vi "DCA Initialize Test.vi"(0 "Instruments to Use":T9, 1 "Files Found?":bool=TRUE, 5 "Seq Count":u32, 9 "Test Parameters In":T10={"Stimulus"={"Use Instrument"=FALSE, "Normalize"=FALSE, "Blank Screen"=FALSE, "Measurement Type"=enum."Voltage DC", "Range"=enum."Auto", "Resolution"=enum."Auto"}, "Measurement"={"Topology"=enum."PI-Network", "Lock Topology"=FALSE, "ATTN Calc"=enum."Power", "Zo"=50.0}, "Limits"=[], "Normalization"={"Normalized?"=FALSE, "Rab Value"=0.0, "Rac Value"=0.0, "Rbc Value"=0.0}}, 11 "error in (no error)":errorcluster) -> (3 "Saved Instrument Configurations":cluster{"DMM Stimulus":T6, "SWI Position":T7}, 4 "Instrument IDs":T5, 6 "Next Action":string, 10 "Test Parameters Out":T10={"Stimulus"={"Use Instrument"=FALSE, "Normalize"=FALSE, "Blank Screen"=FALSE, "Measurement Type"=enum."Voltage DC", "Range"=enum."Auto", "Resolution"=enum."Auto"}, "Measurement"={"Topology"=enum."PI-Network", "Lock Topology"=FALSE, "ATTN Calc"=enum."Power", "Zo"=50.0}, "Limits"=[], "Normalization"={"Normalized?"=FALSE, "Rab Value"=0.0, "Rac Value"=0.0, "Rbc Value"=0.0}}, 12 "Calibration":T1, 14 "Driver Refs":T4, 15 "error out":errorcluster {"code" format="%.0x"})   [LabVIEW 2011]
uses:
  TypeDefs/DCA Test Parameters.ctl
  TypeDefs/DCA Stimulus Parameters.ctl
  TypeDefs/DCA Measurement Cluster.ctl
  TypeDefs/DCA Topology.ctl
  TypeDefs/DCA Attenuation Calculation.ctl
  TypeDefs/DCA Limit.ctl
  TypeDefs/DCA Limit Quantity.ctl
  TypeDefs/DCA Limit Comparison.ctl
  TypeDefs/DCA Limit Operation.ctl
  Test Referential Limit.ctl
  TypeDefs/DCA Calibration State.ctl
  server/database/Stations/Instruments/Instrument Record.ctl
  drivers/SWI/Sea-Level/TypeDefs/Sea-Level SWI Position.ctl
  drivers/DMM/DMM Driver Ref.ctl
  drivers/SWI/SWI Driver Ref.ctl
  drivers/DMM/DMM Command.ctl
  drivers/SWI/SWI Command.ctl
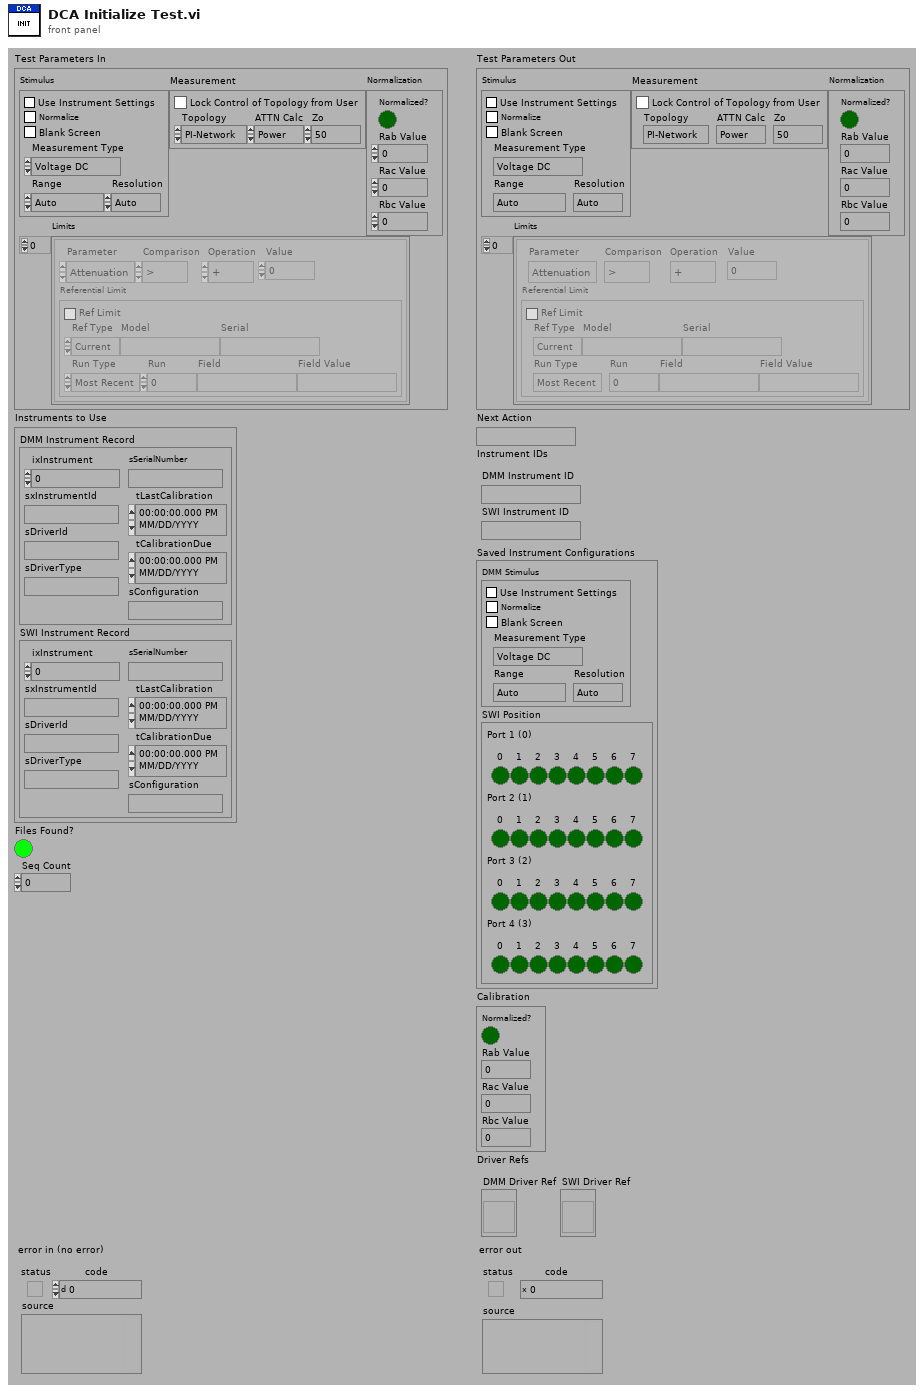
[diagram p1: front panel]
types:
  T1 = typedef "DCA Calibration State.ctl" = cluster{"Normalized?":bool, "Rab Value":dbl, "Rac Value":dbl, "Rbc Value":dbl}
  T2 = typedef "DMM Driver Ref.ctl" = refnum<vi>
  T3 = typedef "SWI Driver Ref.ctl" = refnum<vi>
  T4 = cluster{"DMM Driver Ref":T2, "SWI Driver Ref":T3}
  T5 = cluster{"DMM Instrument ID":string, "SWI Instrument ID":string}
  T6 = typedef "DCA Stimulus Parameters.ctl" = cluster{"Use Instrument":bool, "Normalize":bool, "Blank Screen":bool, "Measurement Type":enum16{"Voltage DC", "Voltage DC Ratio", "Voltage AC", "Current DC", "Current AC", "Resistance", "Fresistance", "Frequency", "Period", "Continuity", "Diode"}, "Range":enum16{"Auto", "Minimum", "Maximum", "100", "1,000", "10,000", "100,000", "1,000,000", "10,000,000", "100,000,000"}, "Resolution":enum16{"Auto", "4 1/2", "5 1/2", "6 1/2"}}
  T7 = typedef "Sea-Level SWI Position.ctl" = cluster{"Port 1 (0)":cluster{"0":bool, "1":bool, "2":bool, "3":bool, "4":bool, "5":bool, "6":bool, "7":bool}, "Port 2 (1)":cluster{"0":bool, "1":bool, "2":bool, "3":bool, "4":bool, "5":bool, "6":bool, "7":bool}, "Port 3 (2)":cluster{"0":bool, "1":bool, "2":bool, "3":bool, "4":bool, "5":bool, "6":bool, "7":bool}, "Port 4 (3)":cluster{"0":bool, "1":bool, "2":bool, "3":bool, "4":bool, "5":bool, "6":bool, "7":bool}}
  T8 = typedef "Instrument Record.ctl" = cluster{"ixInstrument":i32, "sxInstrumentId":string, "sDriverId":string, "sDriverType":string, "sSerialNumber":string, "tLastCalibration":timestamp, "tCalibrationDue":timestamp, "sConfiguration":string}
  T9 = cluster{"DMM Instrument Record":T8, "SWI Instrument Record":T8}
  T10 = typedef "DCA Test Parameters.ctl" = cluster{"Stimulus":T6, "Measurement":T11, "Limits":T14[], "Normalization":T1}
  T11 = typedef "DCA Measurement Cluster.ctl" = cluster{"Topology":T12, "Lock Topology":bool, "ATTN Calc":T13, "Zo":dbl}
  T12 = typedef "DCA Topology.ctl" = enum32{"PI-Network", "T-Network"}
  T13 = typedef "DCA Attenuation Calculation.ctl" = enum32{"Power", "Voltage"}
  T14 = typedef "DCA Limit.ctl" = cluster{"Parameter":T15, "Comparison":T16, "Operation":T17, "Value":dbl, "Referential Limit":T18}
  T15 = typedef "DCA Limit Quantity.ctl" = enum16{"Attenuation", "Zin", "Zout", "R1", "R2", "R3", "Rab", "Rac", "Rbc"}
  T16 = typedef "DCA Limit Comparison.ctl" = enum16{">", ">=", "<", "<="}
  T17 = typedef "DCA Limit Operation.ctl" = enum16{"+", "-"}
  T18 = typedef "Test Referential Limit.ctl" = cluster{"Ref Limit":bool, "Ref Type":enum16{"Current", "Specify"}, "Model":string, "Serial":string, "Run Type":enum16{"Most Recent", "Run #", "Match Field"}, "Run":i32, "Field":string, "Field Value":string}
  T19 = enum16{"Voltage DC", "Voltage DC Ratio", "Voltage AC", "Current DC", "Current AC", "Resistance", "Fresistance", "Frequency", "Period", "Continuity", "Diode"}
  T20 = typedef "DMM Command.ctl" = enum16{"LOAD", "INITIALIZE", "PRESET", "GET STIMULUS", "SET STIMULUS", "MEASURE", "RELEASE", "UNLOAD", "GET CALIBRATION", "CALIBRATE"}
  T21 = typedef "SWI Command.ctl" = enum16{"LOAD", "INITIALIZE", "PRESET", "SET STIMULUS", "GET STIMULUS", "GET INFO", "RELEASE", "UNLOAD"}
  T22 = cluster{"DMM Flat Output":string, "SWI Flat Output":string}
  T23 = cluster{"dup Drv Refnum":T2, "dup Drv Refnum":T3}
  T24 = typedef "DCA Dialog Response.ctl" = enum16{"None", "Normalize", "Ignore", "Abort", "Abort All"}
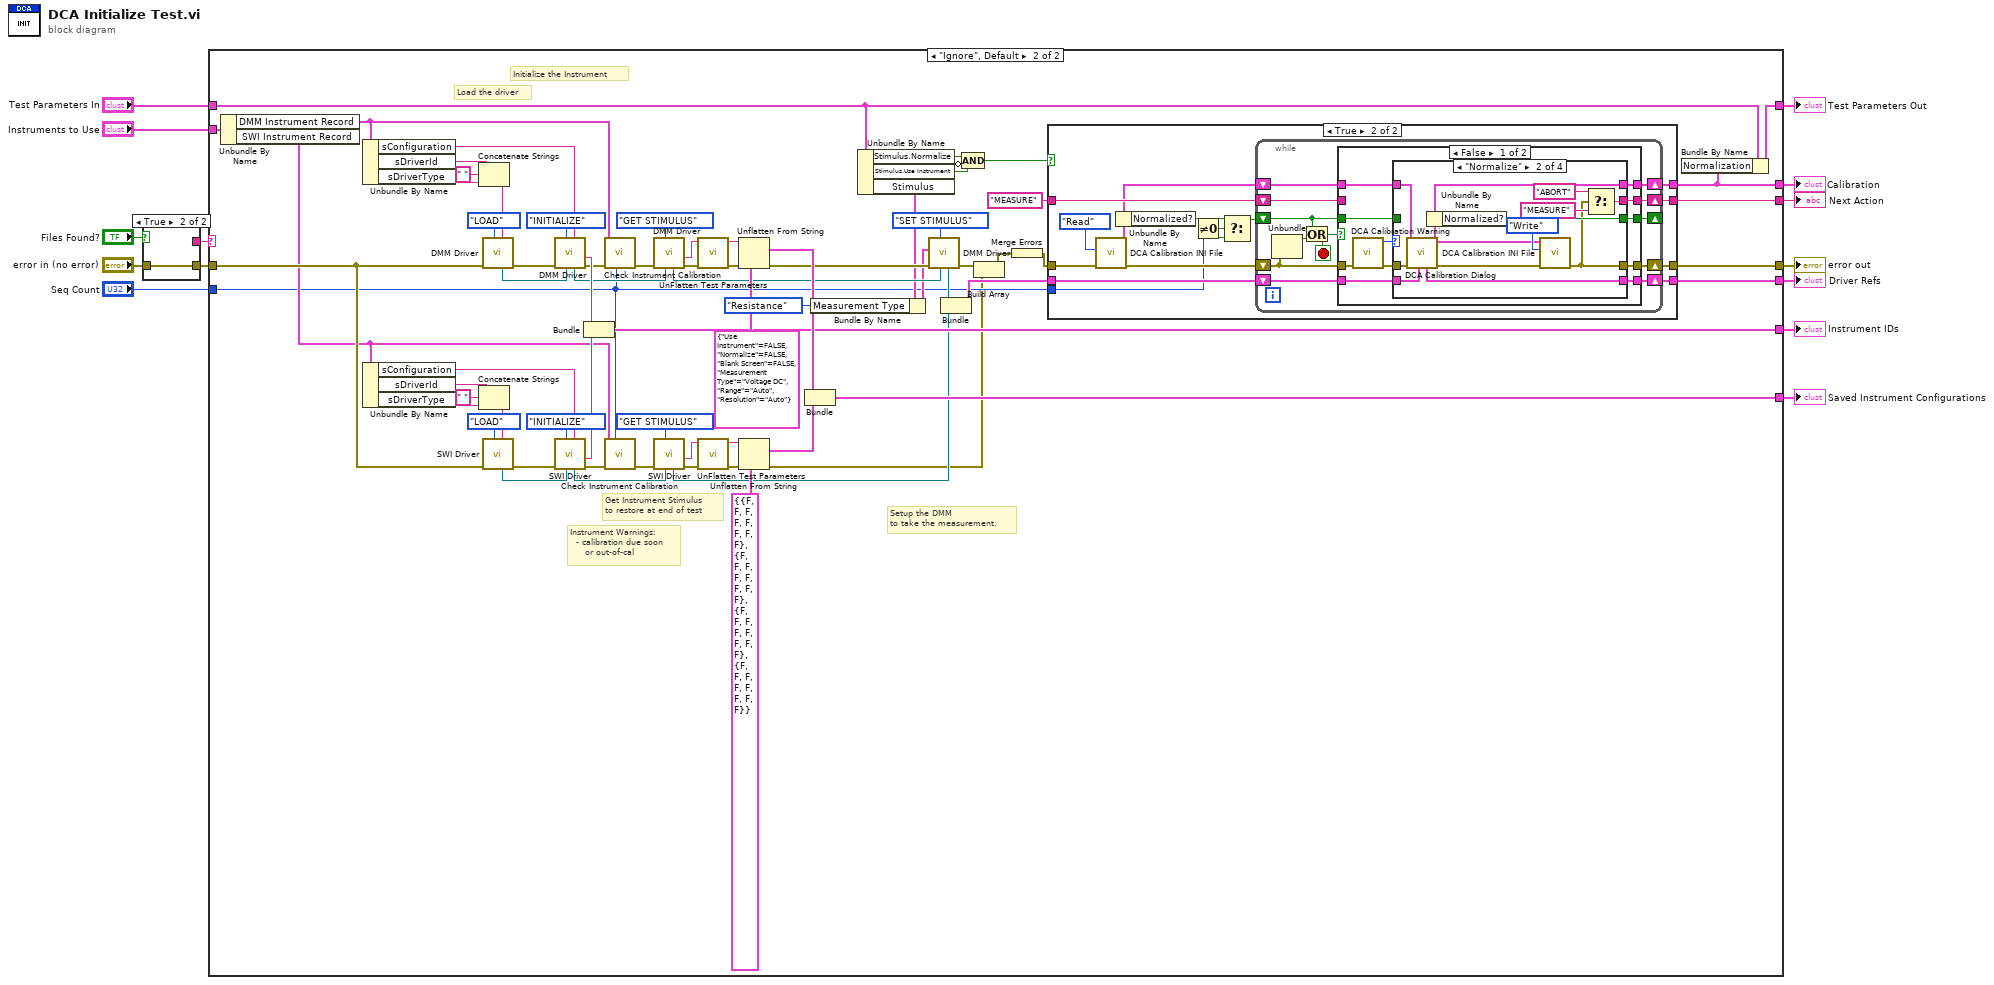
[diagram p0: block diagram]
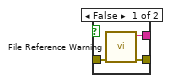
[diagram p2: hidden frame]
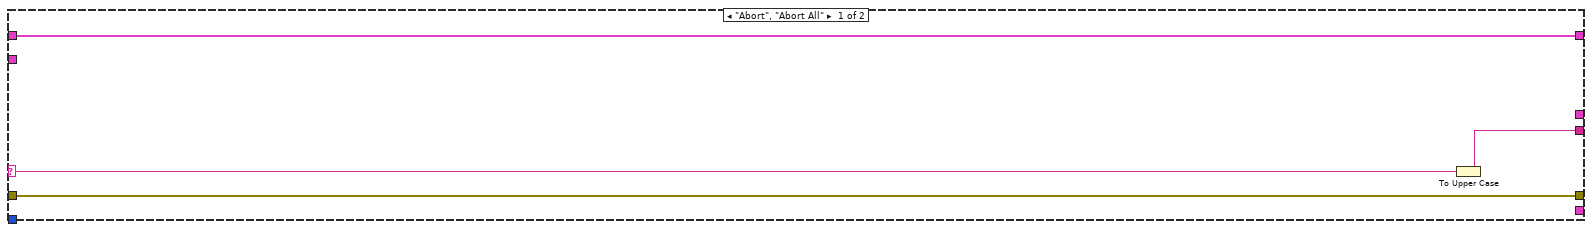
[diagram p3: hidden frame]
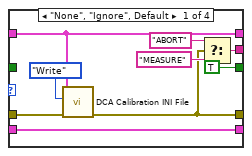
[diagram p5: hidden frame]
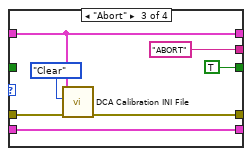
[diagram p6: hidden frame]
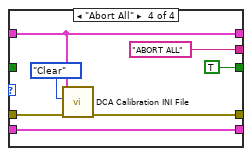
[diagram p7: hidden frame]
diagram:
  n1 = case shown="True" "Files Found?" {
    tunnel: "error in (no error)" -> [w17 w18]
    tunnel: [w16 w18] -> w4
    tunnel: [w15 _] -> w3
    frame False {
      n2 = call "File Reference Warning.vi"("error in (no error)"=w17) -> ("error out"=w16:errorcluster, "Command"=w15:string)  [unwired: 9 out]
    }
    frame True {
    }
  }
  n3 = case shown="\"Ignore\", Default" w3 {
    selector: w3 -> [w20 _]
    tunnel: "Test Parameters In" -> [w21 w27]
    tunnel: w4 -> [w22 w75]
    tunnel: [_ w59] -> w13
    tunnel: [_ w28] -> w12
    tunnel: [_ w56] -> w11
    tunnel: "Instruments to Use" -> [_ w55]
    tunnel: [w19 w50] -> w9
    tunnel: [w22 w41] -> w8
    tunnel: [_ w25] -> w7
    tunnel: [w21 w26] -> w2
    tunnel: "Seq Count" -> [_ w24]
    frame "Abort", "Abort All" {
      n4 = To Upper Case(1:w20) -> (0:w19:string)
    }
    frame "Ignore", Default {
      # "Setup the DMM\nto take the measurement."
      # "Instrument Warnings:\n  - calibration due soon\n     or out-of-cal"
      # "Get Instrument Stimulus\nto restore at end of test"
      # "Initialize the Instrument"
      # "Load the driver"
      n5 = Unbundle By Name(w55) -> ("DMM Instrument Record"=w54:T8, "SWI Instrument Record"=w53:T8)
      n6 = Unbundle By Name(w54) -> ("sConfiguration"=w85:string, "sDriverId"=w84:string, "sDriverType"=w88:string)
      n7 = Unbundle By Name(w53) -> ("sConfiguration"=w81:string, "sDriverId"=w82:string, "sDriverType"=w78:string)
      n8 = Concatenate Strings(w84, " " ("string"), w88) -> (w87:string)
      n9 = Concatenate Strings(w82, " " ("string"), w78) -> (w79:string)
      n10 = call "DMM Driver.vi"("DMM Configuration (\"\")"=w87, "DMM Command"=DMM_Command."LOAD" ("VNA Command"), "error in (no error)"=w75) -> ("error out"=w89:errorcluster, "dup Drv Refnum"=w47:T2)  [unwired: 2 in, 5 out]
      n11 = call "SWI Driver.vi"("SWI Configuration (\"\")"=w79, "SWI Command"=SWI_Command."LOAD", "error in (no error)"=w75) -> ("error out"=w74:errorcluster, "dup Drv Refnum"=w49:T3)  [unwired: 2 in, 5 out]
      n12 = call "DMM Driver.vi"("DMM Configuration (\"\")"=w85, "Drv Refnum"=w47, "DMM Command"=DMM_Command."INITIALIZE" ("VNA Command"), "error in (no error)"=w89) -> ("error out"=w51:errorcluster, "DMM Flat Output"=w58:string, "dup Drv Refnum"=w45:T2)  [unwired: 1 in, 4 out]
      n13 = call "SWI Driver.vi"("SWI Configuration (\"\")"=w81, "Drv Refnum"=w49, "SWI Command"=SWI_Command."INITIALIZE", "error in (no error)"=w74) -> ("error out"=w52:errorcluster, "SWI Flat Output"=w57:string, "dup Drv Refnum"=w48:T3)  [unwired: 1 in, 4 out]
      n14 = Bundle("DMM Flat Output"=w58, "SWI Flat Output"=w57) -> (w56:T22)  [unwired: 1 out]
      n15 = call "Check Instrument Calibration.vi"("Seq Count"=w24, "error in (no error)"=w51, "Instrument Record"=w54) -> ("error out"=w83:errorcluster)  [unwired: 1 in, 7 out]
      n16 = call "Check Instrument Calibration.vi"("Seq Count"=w24, "error in (no error)"=w52, "Instrument Record"=w53) -> ("error out"=w73:errorcluster)  [unwired: 1 in, 7 out]
      n17 = call "DMM Driver.vi"("Drv Refnum"=w45, "DMM Command"=DMM_Command."GET STIMULUS" ("VNA Command"), "error in (no error)"=w83) -> ("error out"=w69:errorcluster, "DMM Flat Output"=w70:string, "dup Drv Refnum"=w46:T2)  [unwired: 2 in, 4 out]
      n18 = call "SWI Driver.vi"("Drv Refnum"=w48, "SWI Command"=SWI_Command."GET STIMULUS", "error in (no error)"=w73) -> ("error out"=w68:errorcluster, "SWI Flat Output"=w67:string, "dup Drv Refnum"=w31:T3)  [unwired: 2 in, 4 out]
      n19 = call "UnFlatten Test Parameters.vi"("error in (no error)"=w69, "Flattened Test Parameters with Version (\"\")"=w70) -> ("error out"=w36:errorcluster, "Flat Test Parameters"=w66:string)  [unwired: 4 out]
      n20 = call "UnFlatten Test Parameters.vi"("error in (no error)"=w68, "Flattened Test Parameters with Version (\"\")"=w67) -> ("error out"=w23:errorcluster, "Flat Test Parameters"=w65:string)  [unwired: 4 out]
      n21 = Unflatten From String(type=T6 {"Use Instrument"=FALSE, "Normalize"=FALSE, "Blank Screen"=FALSE, "Measurement Type"=enum."Voltage DC", "Range"=enum."Auto", "Resolution"=enum."Auto"} ("DMM Stimulus"), binary string=w66, error in (no error)=w36) -> (value=w60:T6, error out=w35:errorcluster)  [unwired: 3 out]
      n22 = Unflatten From String(type=T7 {"Port 1 (0)"={"0"=FALSE, "1"=FALSE, "2"=FALSE, "3"=FALSE, "4"=FALSE, "5"=FALSE, "6"=FALSE, "7"=FALSE}, "Port 2 (1)"={"0"=FALSE, "1"=FALSE, "2"=FALSE, "3"=FALSE, "4"=FALSE, "5"=FALSE, "6"=FALSE, "7"=FALSE}, "Port 3 (2)"={"0"=FALSE, "1"=FALSE, "2"=FALSE, "3"=FALSE, "4"=FALSE, "5"=FALSE, "6"=FALSE, "7"=FALSE}, "Port 4 (3)"={"0"=FALSE, "1"=FALSE, "2"=FALSE, "3"=FALSE, "4"=FALSE, "5"=FALSE, "6"=FALSE, "7"=FALSE}} ("SWI Stimulus"), binary string=w65, error in (no error)=w23) -> (value=w61:T7)  [unwired: 4 out]
      n23 = Bundle("DMM Stimulus"=w60, "SWI Stimulus"=w61) -> (w59:cluster{"DMM Stimulus":T6, "SWI Stimulus":T7})  [unwired: 1 out]
      n24 = Unbundle By Name(w27) -> ("Stimulus.Normalize"=w39:bool, "Stimulus.Use Instrument"=w37:bool, "Stimulus"=w33:T6)
      n25 = Bundle By Name(cluster=w33, "Measurement Type"=T19."Resistance") -> (w32:T6)
      n26 = call "DMM Driver.vi"("Drv Refnum"=w46, "DMM Command"=DMM_Command."SET STIMULUS" ("VNA Command"), "error in (no error)"=w35, "DMM Stimulus"=w32) -> ("error out"=w43:errorcluster, "dup Drv Refnum"=w30:T2)  [unwired: 3 in, 3 out]
      n27 = Bundle("dup Drv Refnum"=w30, "dup Drv Refnum"=w31) -> (w29:T23)  [unwired: 1 out]
      n28 = Compound Arithmetic op=AND(w39, invert w37) -> (w38:bool)
      n29 = Build Array(w43, w23) -> (w62:errorcluster[])
      n30 = Merge Errors(w62) -> (w42:errorcluster)
      n31 = case shown="True" w38 {
        tunnel: w42 -> [w94 w102]
        tunnel: [w94 w108] -> w41
        tunnel: [w92 w107] -> w50
        tunnel: w29 -> [w93 w103]
        tunnel: [w93 w106] -> w28
        tunnel: "MEASURE" ("Next Action") -> [w92 w105]
        tunnel: [_ w104] -> w25
        tunnel: w24 -> [_ w99]
        frame False {
        }
        frame True {
          n32 = call "DCA Calibration INI File.vi"("error in (no error)"=w102, "Operation"=enum16{"Read", "Write", "Clear"}."Read") -> ("error out"=w101:errorcluster, "Calibration Out"=w100:T1)  [unwired: 1 in, 7 out]
          n33 = Unbundle By Name(w100) -> ("Normalized?"=w98:bool)
          n34 = Not Equal To 0?(x=w99) -> (x != 0?=w97:bool)
          n35 = Select(t=w98, s=w97, f=w97) -> (s? t:f=w96:bool)
          n36 = while {
            shift-right: [w119] -> w108
            shift-left: w101 -> [w118]
            shift-right: [w114] -> _
            shift-left: w96 -> [w117]
            shift-right: [w112] -> w106
            shift-left: w103 -> [w113]
            shift-right: [w115] -> w107
            shift-left: w105 -> [w111]
            shift-right: [w109] -> w104
            shift-left: w100 -> [w110]
            stop <- w116 stop-if-true
            n37 = Unbundle(w118) -> ("status"=w120:bool)  [unwired: 2 out]
            n38 = Or(x=w117, y=w120) -> (x .or. y?=w116:bool)
            n39 = case shown="False" w116 {
              tunnel: w118 -> [w131 w171]
              tunnel: [w127 w171] -> w119
              tunnel: w117 -> [w125 w170]
              tunnel: [w129 w168] -> w115
              tunnel: [w126 w170] -> w114
              tunnel: w113 -> [w124 w169]
              tunnel: [w123 w169] -> w112
              tunnel: w111 -> [_ w168]
              tunnel: w110 -> [w122 w167]
              tunnel: [w121 w167] -> w109
              frame False {
                n40 = call "DCA Calibration Warning.vi"("error in (no error)"=w131) -> ("error out"=w128:errorcluster, "Choice"=w130:T24)  [unwired: 1 in, 4 out]
                n41 = case shown="\"Normalize\"" w130 {
                  tunnel: [w137 w145 "ABORT" "ABORT ALL"] -> w129
                  tunnel: w128 -> [w135 w152 w157 w164]
                  tunnel: [w134 w142 w156 w163] -> w127
                  tunnel: [TRUE ("Calibrated?") w149 TRUE ("Calibrated?") TRUE ("Calibrated?")] -> w126
                  tunnel: w125 -> [_ _ _ _]
                  tunnel: w124 -> [w140 w151 w159 w166]
                  tunnel: [w140 w150 w159 w166] -> w123
                  tunnel: w122 -> [w133 w148 w155 w162]
                  tunnel: [w133 w141 w155 w162] -> w121
                  frame "None", "Ignore", Default {
                    n42 = call "DCA Calibration INI File.vi"("error in (no error)"=w135, "Operation"=enum16{"Read", "Write", "Clear"}."Write", "Calibration In"=w133) -> ("error out"=w134:errorcluster)  [unwired: 8 out]
                    n43 = Select(t="ABORT", s=w134, f="MEASURE") -> (s? t:f=w137:string)
                  }
                  frame "Normalize" {
                    n44 = call "DCA Calibration Dialog.vi"("Driver Refs"=w151, "error in (no error)"=w152, "Current Calibration"=w148) -> ("error out"=w143:errorcluster, "Calibration Out"=w141:T1, "Driver Refs Out"=w150:T4)  [unwired: 6 out]
                    n45 = Unbundle By Name(w141) -> ("Normalized?"=w149:bool)
                    n46 = call "DCA Calibration INI File.vi"("error in (no error)"=w143, "Operation"=enum16{"Read", "Write", "Clear"}."Write", "Calibration In"=w141) -> ("error out"=w142:errorcluster)  [unwired: 8 out]
                    n47 = Select(t="ABORT", s=w142, f="MEASURE") -> (s? t:f=w145:string)
                  }
                  frame "Abort" {
                    n48 = call "DCA Calibration INI File.vi"("error in (no error)"=w157, "Operation"=enum16{"Read", "Write", "Clear"}."Clear", "Calibration In"=w155) -> ("error out"=w156:errorcluster)  [unwired: 8 out]
                  }
                  frame "Abort All" {
                    n49 = call "DCA Calibration INI File.vi"("error in (no error)"=w164, "Operation"=enum16{"Read", "Write", "Clear"}."Clear", "Calibration In"=w162) -> ("error out"=w163:errorcluster)  [unwired: 8 out]
                  }
                }
              }
              frame True {
              }
            }
          }
        }
      }
      n50 = Bundle By Name(cluster=w27, "Normalization"=w25) -> (w26:T10)
    }
  }
  "error out" <- w8
  "Test Parameters Out" <- w2
  "Next Action" <- w9
  "Saved Instrument Configurations" <- w13
  "Instrument IDs" <- w11
  "Driver Refs" <- w12
  "Calibration" <- w7
